vi "Find Property in File Header_Main.vi"() -> ()   [LabVIEW 2018]
panel:
  out "Property Value":string
  in  "Property Name":string
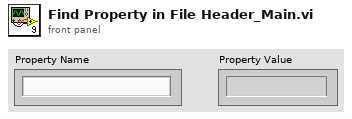
[diagram p1: front panel]
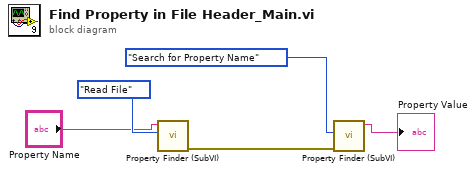
[diagram p0: block diagram]
diagram:
  n1 = call "Property Finder (SubVI).vi"("Enum"=enum16{"Read File", "Search for Property Name"}."Read File", "Property Name"="Property Name") -> ("error out"=w5:errorcluster)  [unwired: 8 in, 1 out]
  n2 = call "Property Finder (SubVI).vi"("error in (no error)"=w5, "Enum"=enum16{"Read File", "Search for Property Name"}."Search for Property Name") -> ("Property Value"=→"Property Value":string)  [unwired: 8 in, 1 out]
